vi "FRTList.vi"(8 "error in (no error)":errorcluster) -> (0 "error out":errorcluster, 3 "FRTList":string[](array[string]))   [LabVIEW 2014]
uses:
  typedefs/ePathsAction.ctl
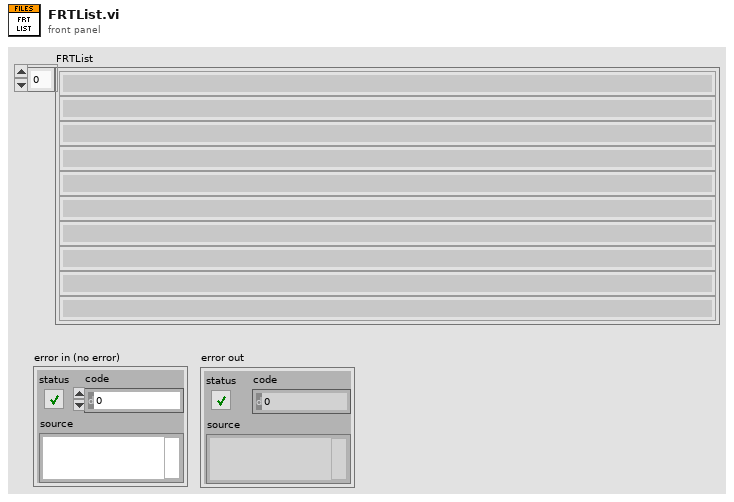
[diagram p1: front panel]
types:
  T1 = typedef "ePathsAction.ctl" = enum16{"Set", "Get", "Load", "Save", "Default", "Exit"}
  T2 = typedef "Paths.ctl" = cluster{"BasePath":path, "CutPath":path, "LastCutPath":path, "CCSPath":path, "LastCCSPath":path, "ResultsPath":path}
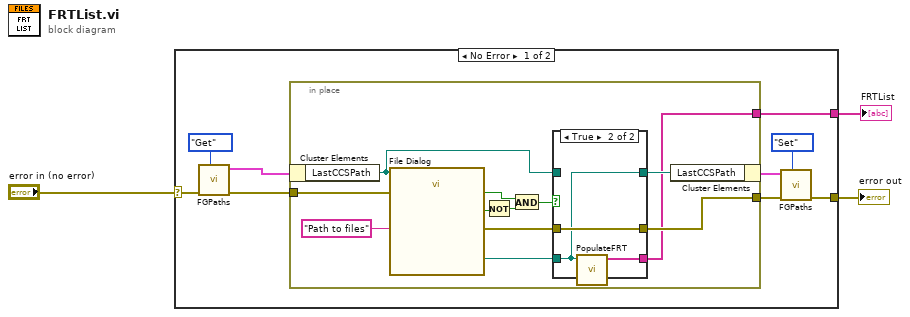
[diagram p0: block diagram]
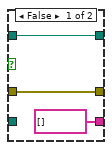
[diagram p2: hidden frame]
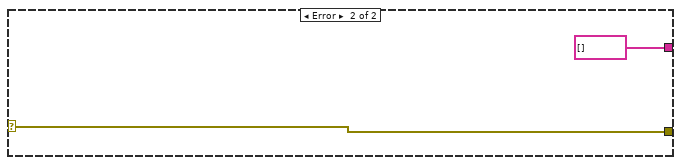
[diagram p3: hidden frame]
diagram:
  n1 = case shown="No Error" "error in (no error)" {
    selector: "error in (no error)" -> [w6 w32]
    tunnel: [w5 w32] -> w2
    tunnel: [w4 string[] [] ("Array")] -> w1
    frame No Error {
      n2 = call "FGPaths.vi"("ePathsAction"=ePathsAction."Get", "error in (no error)"=w6) -> ("error out"=w7:errorcluster, "PathsOut"=w9:T2)  [unwired: 8 in]
      n3 = in-place {
        in-place-border: w7 -> [w17]
        in-place-border: [w14] -> w12
        in-place-border: [w13] -> w4
        n4 = in-place-cluster #1(w9) -> ("LastCCSPath"=w15:path)
        n5 = call "File Dialog"("start path"=w15, "prompt"="Path to files", "error in"=w17) -> ("selected path"=w18:path, "exists"=w21:bool, "cancelled"=w22:bool, "error out"=w19:errorcluster)  [unwired: 9 in]
        n6 = Not(x=w22) -> (.not. x?=w23:bool)
        n7 = And(x=w21, y=w23) -> (x .and. y?=w20:bool)
        n8 = case shown="True" w20 {
          tunnel: w19 -> [w27 w30]
          tunnel: [w27 w30] -> w14
          tunnel: w18 -> [_ w28]
          tunnel: [string[] [] ("Array") w29] -> w13
          tunnel: [w26 w28] -> w16
          tunnel: w15 -> [w26 _]
          frame False {
          }
          frame True {
            n9 = call "PopulateFRT.vi"("Path"=w28) -> ("Array"=w29:string[])  [unwired: 10 in]
          }
        }
        n10 = in-place-cluster #1("LastCCSPath"=w16) -> (w10:T2)
      }
      n11 = call "FGPaths.vi"("ePathsAction"=ePathsAction."Set", "error in (no error)"=w12, "PathsIn"=w10) -> ("error out"=w5:errorcluster)  [unwired: 7 in, 1 out]
    }
    frame Error {
    }
  }
  "error out" <- w2
  "FRTList" <- w1
